vi "Command Editor Dialog 3.vi"(7 "Name(\"\" to use uuid)":string="Event CSM Tiny", 8 "Error in":errorcluster caption="Error in (no error)", 11 "CSM States":string="UI: Front Panel State >> Open -@ abc") -> (0 "Error out":errorcluster, 3 "Command out":string)   [LabVIEW 2017]
uses:
  _Shared/Single-Line Type.ctl
  _Shared/CSM Part Property.ctl
  _Shared/Single-Line Selection Type.ctl
  <vilib>/Utility/miscctls.llb/LVRowAndColumnUnsignedTypeDef.ctl
  AdvanceAPI/CSM - Keywords.vi
  _Support/Common/Trim Single line Text.vi
  AdvanceAPI/CSM - Break Down Multiple States String.vi
  AdvanceAPI/CSM - Compact Multiple States.vi
  _Polymophic/CSM - Filter Duplicated Lines.vi
  Communicable State Machine.lvlib
  _Shared/CSM Shared.lvlib
panel:
  out "MsgType":string
  out "Selction":string
  out "SelType":string
  out "Ref-String":string
  in  "clear arguments":bool
  in  "->|":bool
  in  "->":bool
  in  "-@":bool
  in  "Candidates":i32(listbox)
  # "Flood of Events:\n\nPanel/Pane Size Event\nSlide/Knob... User Event by dragging\nNumeric Control Value Change Event by Arraw Button"
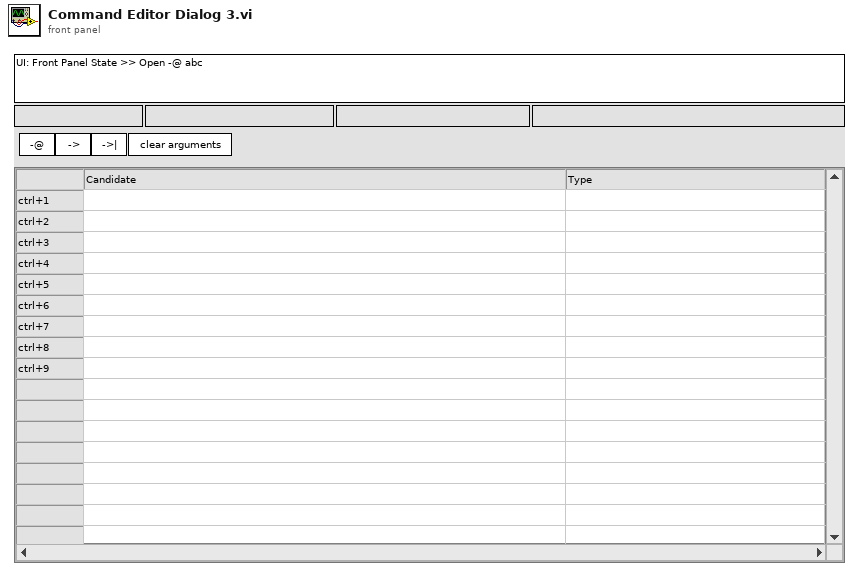
[diagram p1: front panel]
types:
  T1 = enum32{"Invalid", "Standard", "Closed", "Hidden", "Minimized", "Maximized"}
  T2 = enum32{"invalid app kind", "Development System", "Run Time System", "Student Edition", "Embedded LabVIEW", "Evaluation", "Custom"}
  T3 = typedef "LVRowAndColumnUnsignedTypeDef.ctl" = cluster{"Row":u32, "Column":u32}
  T4 = typedef "Communicable State Machine.lvlib/_CSM_Response Source Message.ctl" = cluster{"‘State":string, "’Arguments":string, "’Error":errorcluster}
  T5 = cluster{"Current VI Reference":refnum<vi>, "Close Panel on Exit?":bool}
  T6 = typedef "CSM Shared.lvlib/CSM Part Property.ctl" = cluster{"Section Start":u32, "Section End":u32, "Start":u32, "End":u32, "Section":string, "Core":string, "Sel Type":T7, "Ref-String":string}
  T7 = typedef "CSM Shared.lvlib/Single-Line Selection Type.ctl" = enum16{"<unknown>", "State-StateOrSignal", "State-ArgSymbol", "State-Arg", "Reg-Oper", "Reg-Symbol", "Msg-State", "Msg-Arg", "Msg-ArgSymbol", "Msg-Symbol", "Msg-Module", "Broadcast-Signal", "Broadcast-ArgSymbol", "Broadcast-Arg", "Broadcast-Symbol", "Broadcast-Oper", "Comment-Symbol", "Comment-Content"}
  T8 = typedef "CSM Shared.lvlib/Single-Line Type.ctl" = enum16{"State", "Message", "Broadcast", "Registration"}
  T9 = cluster{"Core":cluster{"Current VI Reference":refnum<vi>, "Close Panel on Exit?":bool}, "CSM States":string, "Selection":T6[], "Msg Type":T8}
  T10 = typedef "LVSelectionTypeDef.ctl" = cluster{"Selection Start":u32, "Selection End":u32}
  T11 = typedef "eventvkey.ctl" = enum16{"ASCII", "Enter", "Return", "Shift", "Ctrl", "Alt", "Cmd", "Opt", "Caps", "NumLock", "Clear", "Break", "Up", "Down", "Left", "Right", "Insert", "Delete", "Home", "End", "PageUp", "PageDown", "Escape", "Help", "Pause", "ScrollLock", "F1", "F2", "F3", "F4", "F5", "F6", "F7", "F8", "F9", "F10", "F11", "F12", "F13", "F14", "F15", "F16", "F17", "F18", "F19", "F20", "F21", "F22", "F23", "F24", "Play", "VolumeUp", "VolumeDown", "Mute", "Two Byte Char"}
  T12 = cluster{"Shift":bool, "Ctrl":bool, "Alt":bool, "Cmd":bool, "Opt":bool}
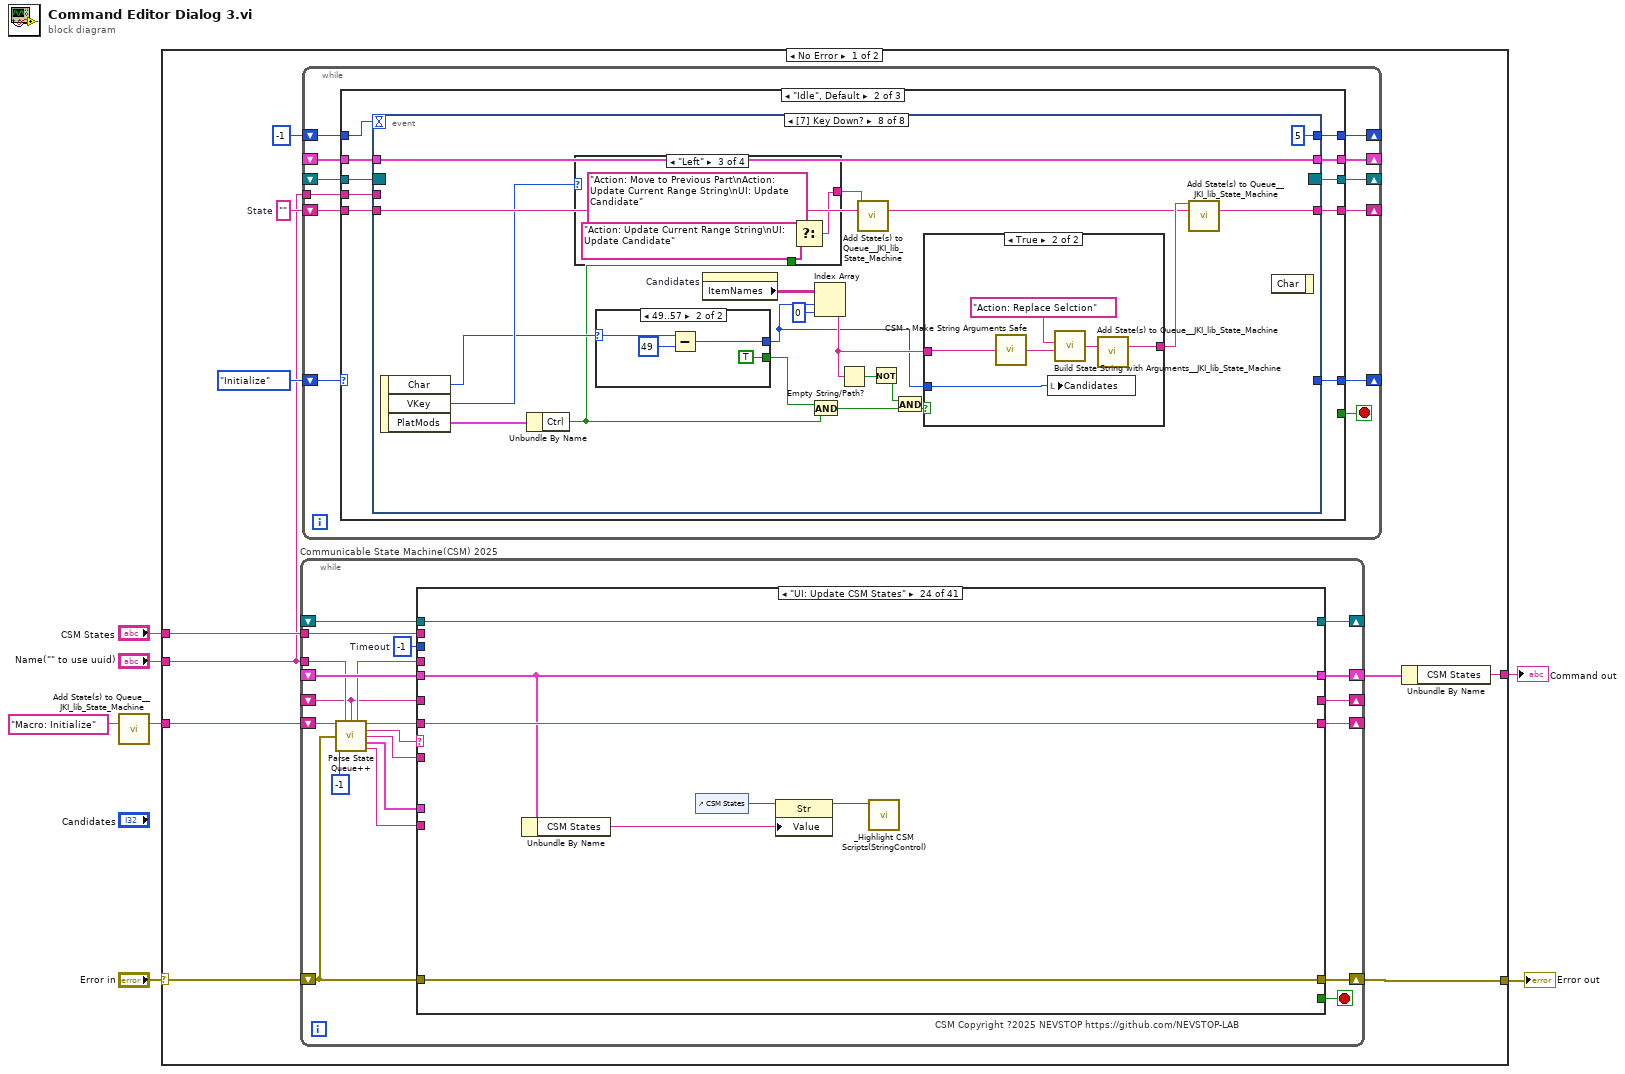
[diagram p0: block diagram]
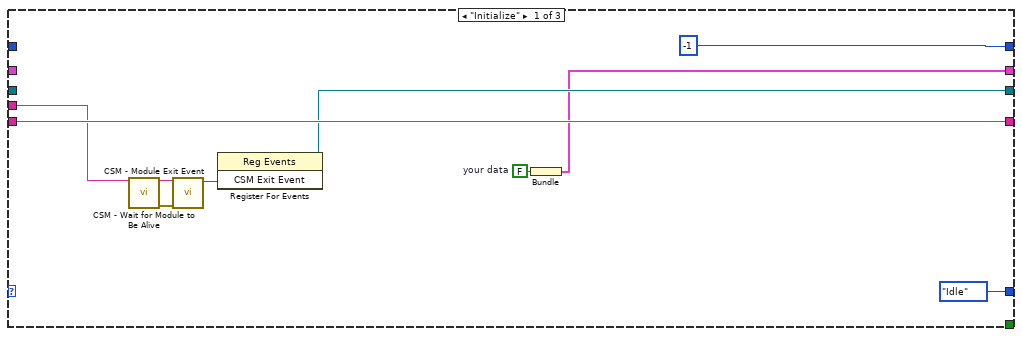
[diagram p2: hidden frame]
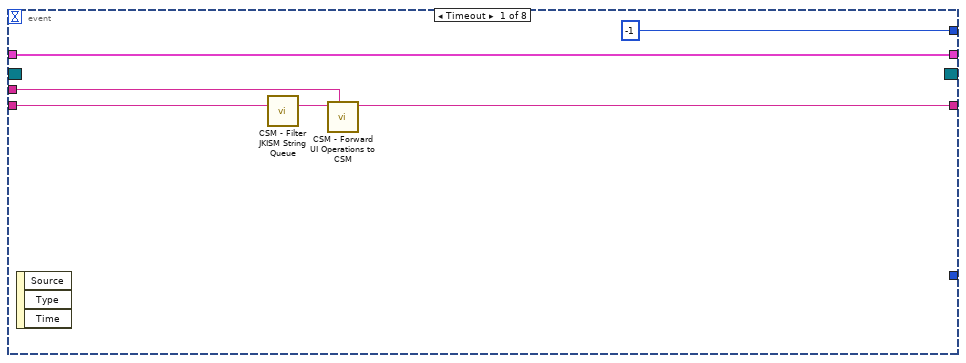
[diagram p3: hidden frame]
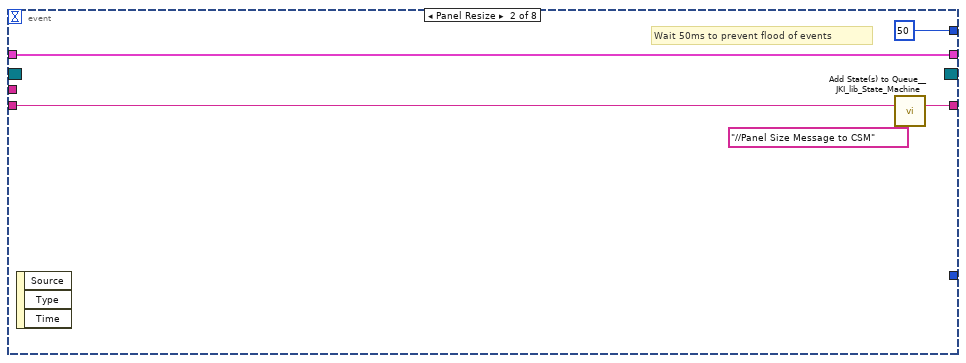
[diagram p4: hidden frame]
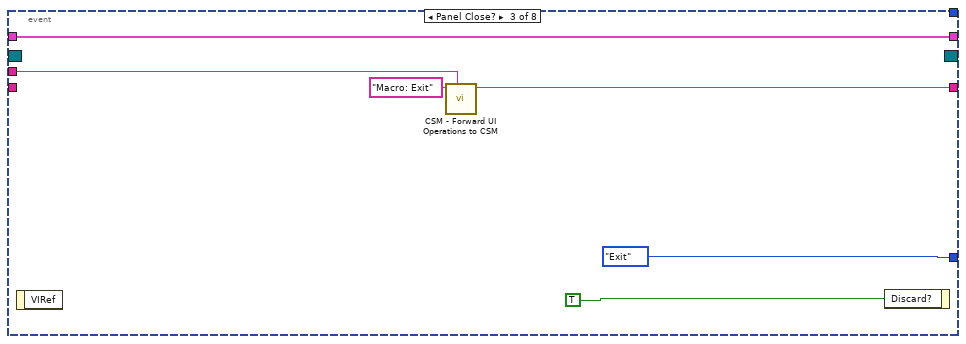
[diagram p5: hidden frame]
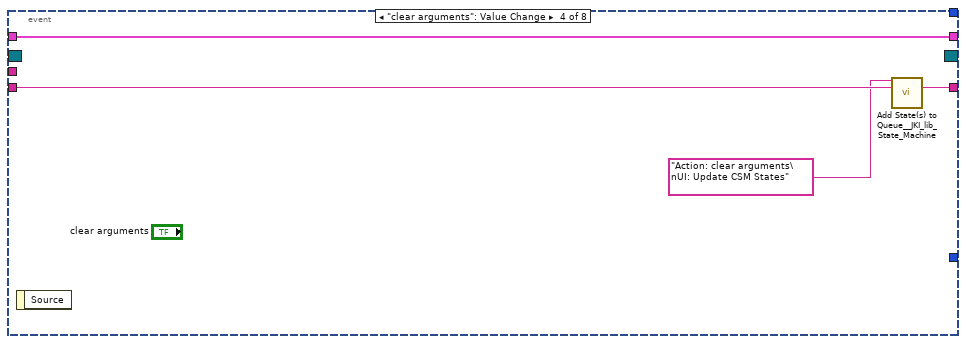
[diagram p6: hidden frame]
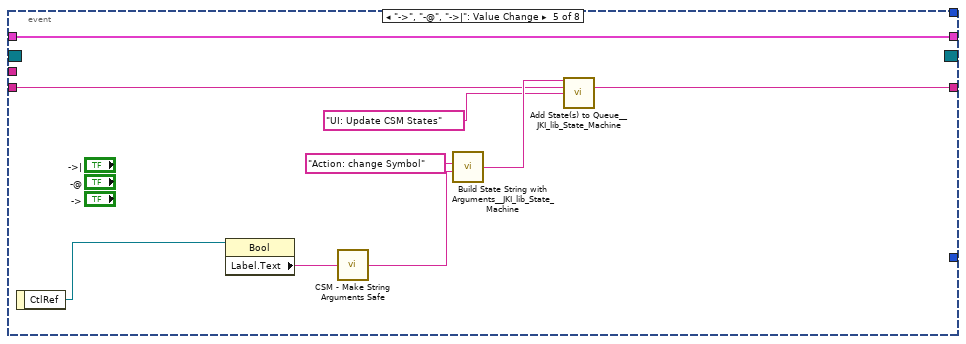
[diagram p7: hidden frame]
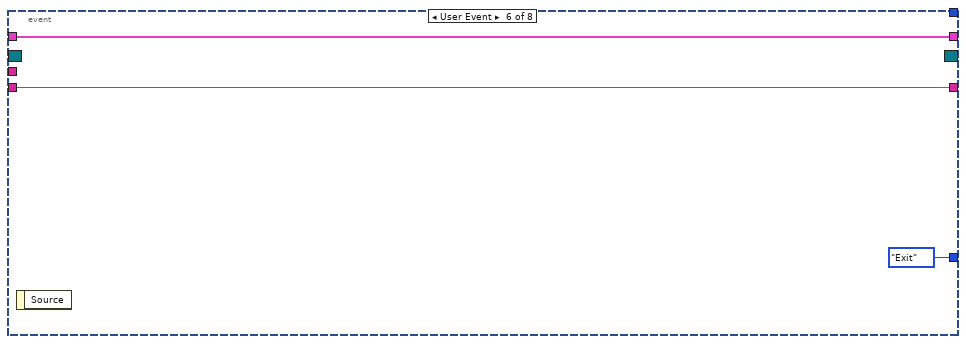
[diagram p8: hidden frame]
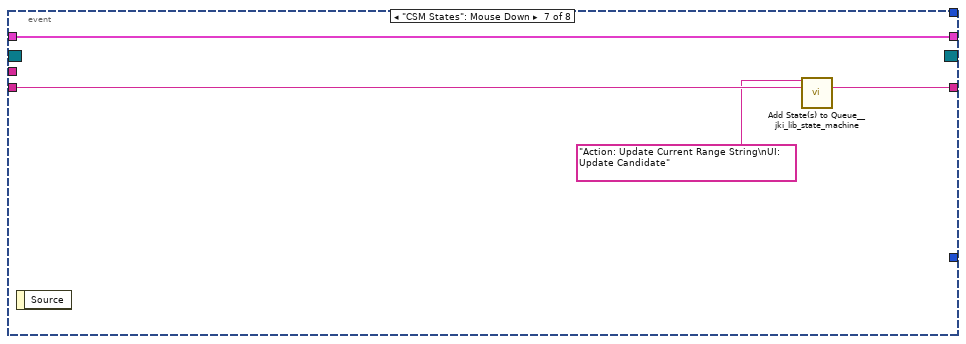
[diagram p9: hidden frame]
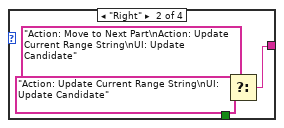
[diagram p11: hidden frame]
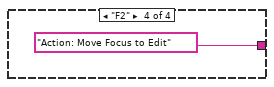
[diagram p12: hidden frame]
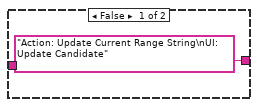
[diagram p13: hidden frame]
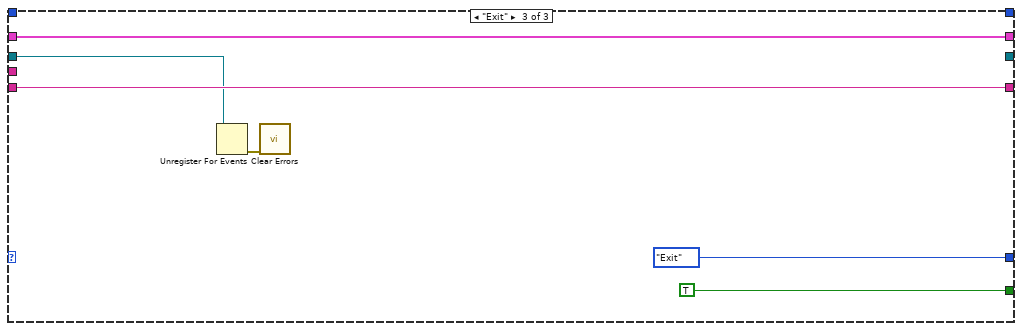
[diagram p15: hidden frame]
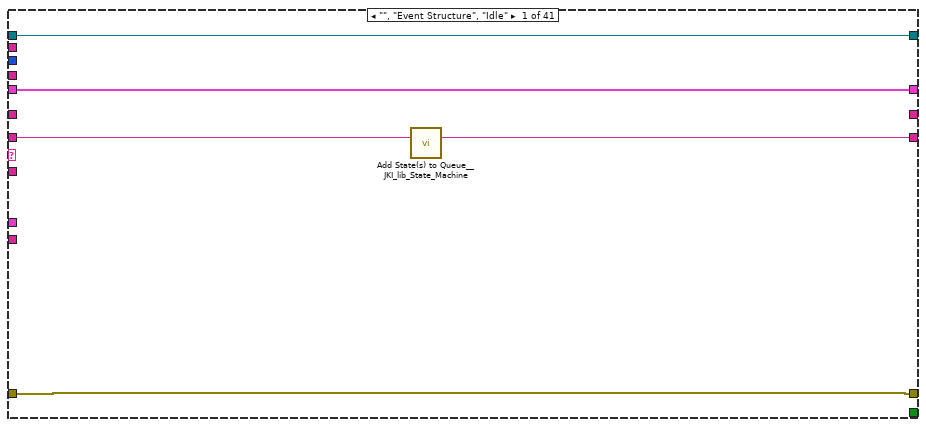
[diagram p16: hidden frame]
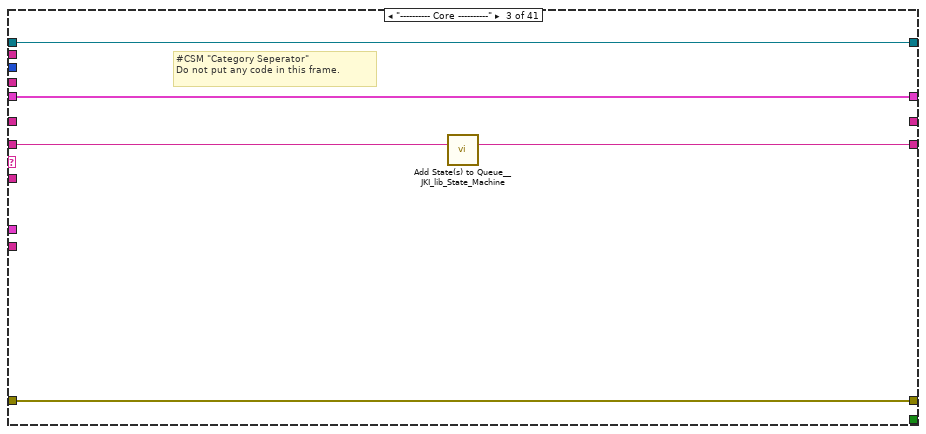
[diagram p18: hidden frame]
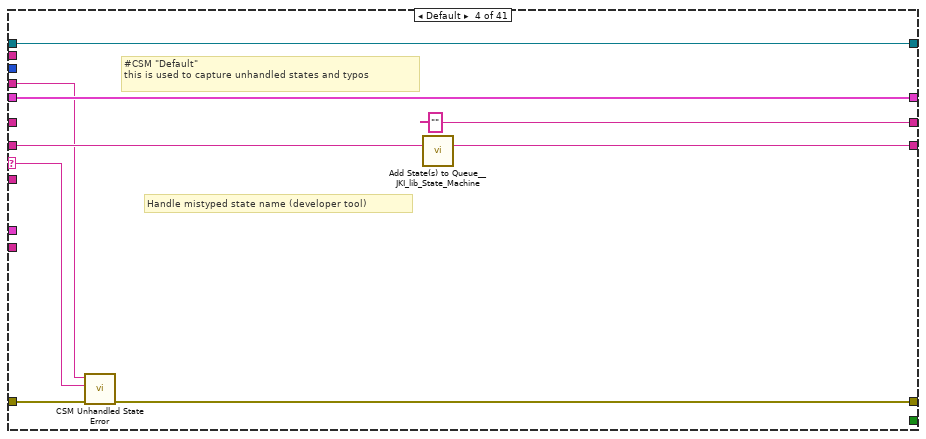
[diagram p19: hidden frame]
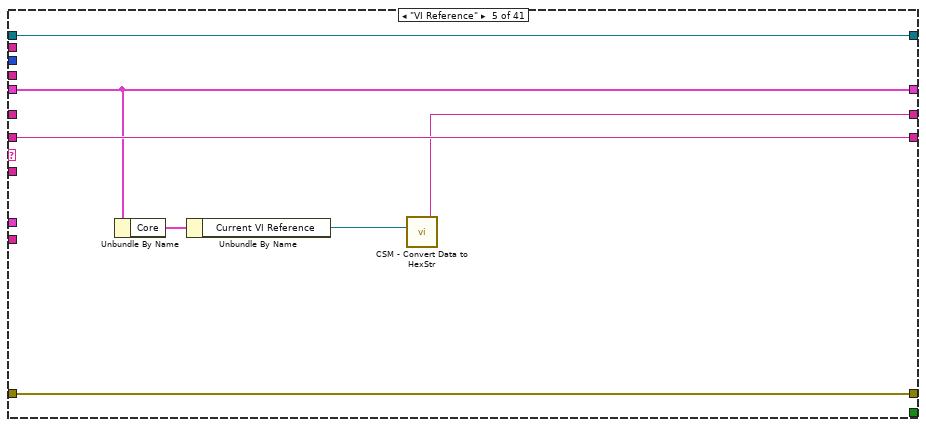
[diagram p20: hidden frame]
diagram:
  n1 = call <vilib>:"Add State(s) to Queue__JKI_lib_State_Machine.vi"("State(s) in (\"\")"="Macro: Initialize" ("Init State(\"Macro: Initialize\")")) -> ("States Out"=w7:string)  [unwired: 14 in]
  n2 = case shown="No Error" "Error in" {
    selector: "Error in" -> [w15 w645]
    tunnel: w7 -> [w17 _]
    tunnel: "Name(\"\" to use uuid)" -> [w8 _]
    tunnel: [w16 w645] -> w4
    tunnel: [w13 w644] -> w1
    tunnel: "CSM States" -> [w9 w644]
    frame No Error {
      w11 = ""  # State
      n3 = while "Communicable State Machine(CSM) 2025" {
        shift-right: [w148] -> w14
        shift-left: _ -> [w147]
        shift-right: [w151] -> w16
        shift-left: w15 -> [w145]
        shift-right: [w150] -> _
        shift-left: w17 -> [w152]
        tunnel: w8 -> [w141]
        shift-right: [w144] -> _
        shift-left: _ -> [w135]
        shift-right: [w143] -> _
        shift-left: _ -> [w142]
        tunnel: w9 -> [w134]
        stop <- w149 stop-if-true
        w146 = -1  # Timeout
        # "CSM Copyright ?2025 NEVSTOP https://github.com/NEVSTOP-LAB"
        n4 = call "Parse State Queue++.vi"("State Queue"=w152, "Name(\"\" to use uuid)"=w141, "Response Arguments"=w135, "Previous Error"=w145, "Dequeue Timeout(0ms)"=-1) -> ("Name Used"=w136:string, "Remaining States"=w153:string, "Current State"=w140:string, "Arguments"=w139:string, ">> Response Source Message >>"=w138:T4, ">> Source CSM >>"=w137:string)  [unwired: 5 in]
        n5 = case shown="\"UI: Update CSM States\"" w140 {
          selector: w140 -> [_ _ _ w170 _ _ _ _ _ _ _ _ _ _ _ _ _ _ _ _ _ _ _ _ _ _ _ _ _ _ _ _ _ _ _ _ _ _ _ _ _]
          tunnel: w153 -> [w154 w161 w167 w175 w182 w188 w211 w217 w224 w233 w246 w261 w267 w272 w281 w288 w293 w300 w304 w310 w318 w329 w345 w416 w420 w424 w435 w449 w455 w467 w470 w473 w485 w494 w514 w542 w571 w588 w593 w602 w627]
          tunnel: w139 -> [_ _ _ _ _ w187 w206 w216 w223 w232 _ _ _ _ _ _ _ _ _ _ _ w324 w339 _ _ _ _ _ _ _ _ w475 _ w486 w504 _ w565 _ _ _ _]
          tunnel: w147 -> [w156 w160 w164 w173 w181 w192 w212 w219 w226 w235 w245 w254 w265 w269 _ w283 w290 w299 w303 w307 w314 w327 w341 w414 w419 w423 w431 w446 w452 w464 w469 w479 w482 w492 w512 w540 w553 w582 w592 w601 w626]
          tunnel: [w157 w162 w165 w168 w183 errorcluster {"status"=FALSE, "code"=0, "source"=""} ("error out") w207 w214 w221 w238 w247 w258 w264 w270 w278 w284 w291 w294 w302 w308 w316 w325 w342 w417 w421 w425 w436 w447 w453 w465 w471 w480 w483 w495 w515 w543 w572 w589 w594 w603 w628] -> w151
          tunnel: w145 -> [w157 w162 w165 w176 w183 w189 w213 w215 w222 _ w247 w258 w264 w270 w278 w285 w291 _ w305 w308 w316 w326 w343 w417 w421 w425 w436 w447 w453 w465 w471 w480 w483 w495 w515 w543 w572 w589 w594 w603 w628]
          tunnel: [w158 w161 w166 w174 w182 w184 w210 w220 w227 w234 w246 w260 w266 w271 w280 w287 w292 w300 w304 w309 w317 w328 w344 w416 w420 w424 w435 w448 w454 w466 w470 w474 w484 w494 w514 w542 w571 w588 w593 w602 w627] -> w150
          tunnel: [_ _ _ _ _ _ TRUE _ _ _ _ _ TRUE _ _ _ _ _ _ _ _ _ _ _ _ _ _ _ _ _ _ _ _ _ _ _ _ _ _ _ _] -> w149
          tunnel: [w156 w160 w164 w173 w181 w192 w212 w219 w226 w236 w245 w259 w265 w269 w279 w283 w290 w299 w303 w307 w314 w327 w341 w414 w419 w423 w431 w446 w452 w464 w469 w477 w482 w489 w509 w537 w569 w581 w592 w601 w626] -> w148
          tunnel: w146 -> [_ _ _ _ _ _ _ _ _ _ _ _ _ _ _ _ _ _ _ _ _ _ _ _ _ _ _ _ _ _ _ _ _ _ _ _ _ _ _ _ _]
          tunnel: w137 -> [_ _ _ _ _ _ _ _ _ w230 _ _ _ _ _ _ _ _ _ _ _ _ _ _ _ _ _ _ _ _ _ _ _ _ _ _ _ _ _ _ _]
          tunnel: w138 -> [_ _ _ _ _ _ _ _ _ w237 _ _ _ _ _ _ _ _ _ _ _ _ _ _ _ _ _ _ _ _ _ _ _ _ _ _ _ _ _ _ _]
          tunnel: [_ _ _ "" w177 _ _ _ _ _ _ _ _ _ _ _ _ _ _ _ _ _ _ _ _ _ _ _ _ _ _ _ _ _ _ _ _ _ _ _ _] -> w144
          tunnel: [w155 w159 w163 w171 w180 w191 w208 w218 w225 w239 w244 w248 w262 w268 w276 w282 w289 w298 w301 w306 w315 w323 w338 w415 w418 w422 w434 w445 w450 w457 w468 w478 w481 w493 w513 w541 w570 w587 w591 w600 w625] -> w143
          tunnel: w142 -> [w155 w159 w163 w171 w180 w191 w208 w218 w225 w239 w244 w248 w262 w268 w276 w282 w289 _ w301 w306 w315 w323 w338 w415 w418 w422 w434 w445 w450 w457 w468 w478 w481 w493 w513 w541 w570 w587 w591 w600 w625]
          tunnel: w136 -> [_ _ _ w169 _ _ w205 _ _ _ _ _ _ _ _ _ _ w297 _ _ _ _ _ _ _ _ _ _ _ _ _ _ _ _ _ _ _ _ _ _ _]
          tunnel: w135 -> [_ _ _ _ _ _ _ _ _ _ _ _ _ _ _ _ _ _ _ _ _ _ _ _ _ _ _ _ _ _ _ _ _ _ _ _ _ _ _ _ _]
          tunnel: w134 -> [_ _ _ _ _ _ _ _ _ _ _ _ _ _ w275 _ _ _ _ _ _ _ _ _ _ _ _ _ _ _ _ _ _ _ _ _ _ _ _ _ _]
          frame "", "Event Structure", "Idle" {
            n6 = call <vilib>:"Add State(s) to Queue__JKI_lib_State_Machine.vi"("State(s) in (\"\")"=w154) -> ("States Out"=w158:string)  [unwired: 14 in]
          }
          frame "CSM Documentation" {
          }
          frame "---------- Core ----------" {
            # "#CSM \"Category Seperator\"\nDo not put any code in this frame."
            n7 = call <vilib>:"Add State(s) to Queue__JKI_lib_State_Machine.vi"("State(s) in (\"\")"=w167) -> ("States Out"=w166:string)  [unwired: 14 in]
          }
          frame Default {
            # "#CSM \"Default\"\nthis is used to capture unhandled states and typos"
            # "Handle mistyped state name (developer tool)"
            n8 = call "CSM Unhandled State Error.vi"("error in (no error)"=w176, "Current State"=w170, "CSM Name"=w169) -> ("error out"=w168:errorcluster)  [unwired: 8 in]
            n9 = call <vilib>:"Add State(s) to Queue__JKI_lib_State_Machine.vi"("State(s) in (\"\")"=w175) -> ("States Out"=w174:string)  [unwired: 14 in]
          }
          frame "VI Reference" {
            n10 = Unbundle By Name(w181) -> ("Core"=w179:T5)
            n11 = Unbundle By Name(w179) -> ("Current VI Reference"=w178:refnum<vi>)
            n12 = call "CSM - Convert Data to HexStr.vi"("Variant"=w178) -> ("HEX String (0-9,A-F)"=w177:string)  [unwired: 8 in]
          }
          frame "Error Handler" {
            # "#CSM Disable this error dialog if you need"
            # "#CSM \"Error Handler\"\nYou can also output any states to clean-up after errors occur"
            # "Clear error"
            n13 = case shown="Error" w189 {
              selector: w189 -> [_ w199]
              tunnel: [w198 w201] -> w185
              tunnel: w188 -> [w198 w200]
              tunnel: w187 -> [w197 _]
              tunnel: [w196 w199] -> w190
              frame No Error {
                n14 = call "CSM - Convert Argument to Error.vi"("Argument"=w197) -> ("error"=w196:errorcluster)  [unwired: 4 in]
                n15 = flat-sequence {
                  frame #0 {
                    # "#CSM External Error Handler Case\nUsually, it's because This CSM register others' \"Error Occurred\" status with \"Error Handler\". If other CSM have any error, the error will be passed here for central handling."
                  }
                }
              }
              frame Error {
                # "#CSM Internal Error Handler Case \nIf any error Occurred, \"Error Occurred\" \nstatus update will be broadcasted to system.\nParameter is Error Cluster."
                n16 = call "CSM - Convert Error to Argument.vi"("error"=w199) -> ("Argument"=w203:string)  [unwired: 4 in]
                n17 = call <vilib>:"Build State String with Arguments__JKI_lib_State_Machine.vi"("Arguments (\"\")"=w203, "State"="Error Occurred" ("Status with Arguments")) -> ("State with Arguments"=w202:string)  [unwired: 4 in]
                n18 = call "CSM - Broadcast Status Change.vi"("Status with Arguments"=w202, "State Queue"=w200) -> ("Remaining States"=w201:string)  [unwired: 13 in]
              }
            }
            n19 = disable-structure shown="Enabled" {
              disable-tunnel: w190 -> [w194 w195]
              frame Enabled {
                n20 = call <vilib>:"General Error Handler.vi"("error in (no error)"=w194) -> ()  [unwired: 10 in, 5 out]
              }
              frame Disabled {
                n21 = call <vilib>:"Clear Errors.vi"("error in (no error)"=w195) -> ()  [unwired: 5 in, 2 out]
              }
            }
            n22 = call <vilib>:"Add State(s) to Queue__JKI_lib_State_Machine.vi"("State(s) in Front (\"\")"="// Post Error States", "State(s) in (\"\")"=w185) -> ("States Out"=w184:string)  [unwired: 13 in]
          }
          frame "Critical Error" {
            # "#CSM Stop in Critical Error\nWhen Critical Error occurs, Stop the loop immediately. Do NOT change this unless you fully understand the impact."
            # "#CSM \"Critical Error\"\nWhen any un-recoverable error occurs, CSM goes into this case."
            n23 = call "CSM Critical Error.vi"("error in (no error)"=w213, "Arugments(as Reason)"=w206, "CSM Name"=w205) -> ("error out"=w207:errorcluster)  [unwired: 8 in]
            n24 = call <vilib>:"Add State(s) to Queue__JKI_lib_State_Machine.vi"("State(s) in (\"\")"=w211) -> ("States Out"=w210:string)  [unwired: 14 in]
          }
          frame "Target Error" {
            # "#CSM \"Target Error\"\nWhen This CSM try to communicate with an un-existed CSM, This CSM goes into this case."
            n25 = call "CSM Target Error.vi"("error in (no error)"=w215, "Arguments(as CSM Name)"=w216) -> ("error out"=w214:errorcluster)  [unwired: 9 in]
            n26 = call <vilib>:"Add State(s) to Queue__JKI_lib_State_Machine.vi"("State(s) in (\"\")"=w217) -> ("States Out"=w220:string)  [unwired: 14 in]
          }
          frame "Target Timeout Error" {
            # "#CSM \"Target Timeout Error\"\nWhen This CSM could not get the sync-call response in time, This CSM goes into this case."
            n27 = call "CSM Target Timeout Error.vi"("error in (no error)"=w222, "Arguments(as CSM Name)"=w223) -> ("error out"=w221:errorcluster)  [unwired: 9 in]
            n28 = call <vilib>:"Add State(s) to Queue__JKI_lib_State_Machine.vi"("State(s) in (\"\")"=w224) -> ("States Out"=w227:string)  [unwired: 14 in]
          }
          frame "Async Response", "Response" {
            n29 = Unbundle(w237) -> ("‘State"=w231:string, "’Arguments"=w229:string, "’Error"=w228:errorcluster)
            n30 = case shown="Default" w231 {
              tunnel: [w243] -> w238
              tunnel: w228 -> [w243]
              tunnel: [w242] -> w236
              tunnel: w235 -> [w242]
              tunnel: [w240] -> w234
              tunnel: w233 -> [w241]
              tunnel: w232 -> [_]
              tunnel: w230 -> [_]
              tunnel: w229 -> [_]
              frame Default {
                # "#CSM Response Comments\nAfter Message is executed, CSM goes to this state for receive the response.\n    For Async Message(->), \"Async Response\" is used. This CSM will goes to \"Async Message Posted\" immediately and receive the \"Async Response\" after the callee finishes the message.\n    For Sync Message(@),  This CSM will wait until the message is done and immediately goes to \"Response\""
                # "#CSM \"Async Response\"\nHandle Async-call Response (\"Async Response\" for ->)"
                # "#CSM \"Response\"\nHandle Sync-call Response (\"Response\" for -@)"
                n31 = call <vilib>:"Add State(s) to Queue__JKI_lib_State_Machine.vi"("State(s) in (\"\")"=w241) -> ("States Out"=w240:string)  [unwired: 14 in]
              }
            }
          }
          frame "Async Message Posted" {
            # "#CSM \"Async Message Posted\"\nAfter Async Message is posted (-> or ->| ), CSM goes to this state for post-action.\nYou can use Argument - State to tell which Async Message is called."
          }
          frame "Initialize Core Data" {
            # "#CSM \"Initialize Core Data\"\nThis is used to determine panel behavior on exit"
            # "originally closed?"
            # "exe?"
            # "If panel starts closed or is an EXE, then close it when we exit"
            n32 = property class="VI"() -> ("FP.State"=w251:T1)  [unwired: 2 in, 2 out]
            n33 = property class="App"() -> ("App.Kind"=w257:T2)  [unwired: 2 in, 2 out]
            n34 = control-ref of="Current VI Reference"() -> (w252:refnum<vi>)
            n35 = Equal?(x=w251, y=T1."Closed" ("Front Panel Window:State")) -> (x = y?=w249:bool)
            n36 = Equal?(x=w257, y=T2."Run Time System" ("Application:Kind")) -> (x = y?=w255:bool)
            n37 = Or(x=w249, y=w255) -> (x .or. y?=w253:bool)
            n38 = Bundle By Name(cluster=w254, "Core.Current VI Reference"=w252, "Core.Close Panel on Exit?"=w253) -> (w259:T9)
            n39 = call <vilib>:"Add State(s) to Queue__JKI_lib_State_Machine.vi"("State(s) in (\"\")"=w261) -> ("States Out"=w260:string)  [unwired: 14 in]
          }
          frame "Exit" {
            # "#CSM \"Exit\"\nCase for exiting the loop. No errors that occur here will be handled."
            n40 = call <vilib>:"Add State(s) to Queue__JKI_lib_State_Machine.vi"("State(s) in (\"\")"=w267) -> ("States Out"=w266:string)  [unwired: 14 in]
          }
          frame "---------- Data ----------" {
            # "#CSM \"Category Seperator\"\nDo not put any code in this frame."
            n41 = call <vilib>:"Add State(s) to Queue__JKI_lib_State_Machine.vi"("State(s) in (\"\")"=w272) -> ("States Out"=w271:string)  [unwired: 14 in]
          }
          frame "Data: Initialize" {
            w273 = T6[] []  # Selection
            w274 = Single-Line_Type."Registration"  # Msg Type
            w277 = T5 {"Current VI Reference"=refnum, "Close Panel on Exit?"=FALSE}  # Core
            n42 = call <vilib>:"Add State(s) to Queue__JKI_lib_State_Machine.vi"("State(s) in (\"\")"=w281) -> ("States Out"=w280:string)  [unwired: 14 in]
            n43 = Bundle("Core"=w277, "CSM States"=w275, "Selection"=w273, "Msg Type"=w274) -> (w279:T9)  [unwired: 1 in]
          }
          frame "Data: Cleanup" {
            # "Cleanup any data and references, here.\n(this is called automatically, by the Macro: Exit)"
            n44 = Unbundle By Name(w283) -> ("Core.Current VI Reference"=w286:refnum<vi>)
            n45 = Close Reference(reference=w286, error in (no error)=w285) -> (error out=w284:errorcluster)
            n46 = call <vilib>:"Add State(s) to Queue__JKI_lib_State_Machine.vi"("State(s) in (\"\")"=w288) -> ("States Out"=w287:string)  [unwired: 14 in]
          }
          frame "---------- Events ----------" {
            # "#CSM \"Category Seperator\"\nDo not put any code in this frame."
            n47 = call <vilib>:"Add State(s) to Queue__JKI_lib_State_Machine.vi"("State(s) in (\"\")"=w293) -> ("States Out"=w292:string)  [unwired: 14 in]
          }
          frame "Events: Register" {
            # "#CSM \"Events: Register\"\nRegister user event. New Message Event is registered to break CSM waiting in event structure by default."
            # "#CSM Register New Message Event\nRegister message event to break Waiting in Event structure."
            n48 = call "CSM - Get New State Notifier Event.vi"("Name(\"\" to use uuid) in"=w297) -> ("Error out"=w295:errorcluster, "New State Notifier Event"=w296:refnum<user-event>)  [unwired: 9 in]
            n49 = register-events(error in=w295, w296) -> (reference out=w298:refnum<event-registration>, error out=w294:errorcluster)  [unwired: 1 in]
          }
          frame "Events: Unregister" {
            # "#CSM \"Events: Unregister\"\nUnregister user event."
            n50 = Unregister For Events(event registration refnum=w301, error in=w305) -> (error out=w302:errorcluster)
          }
          frame "---------- UI ----------" {
            # "#CSM \"Category Seperator\"\nDo not put any code in this frame."
            n51 = call <vilib>:"Add State(s) to Queue__JKI_lib_State_Machine.vi"("State(s) in (\"\")"=w310) -> ("States Out"=w309:string)  [unwired: 14 in]
          }
          frame "UI: Initialize" {
            n52 = for {
              N: 9 -> [_]
              tunnel: [w320] -> w312 mode=indexing
              i -> [w322]
              n53 = Increment(x=w322) -> (x+1=w319:i32)
              n54 = Format Into String(format string="ctrl+%d", w319) -> (resulting string=w320:string)  [unwired: 2 in, 1 out]
            }
            n55 = property on="Candidates" class="MCListbox (strict)"("RowHdrs[]"=w312, "TopLeft"=T3 {"Row"=0, "Column"=0} ("Top Left Visible Cell")) -> ()  [unwired: 2 in, 2 out]
            n56 = call <vilib>:"Add State(s) to Queue__JKI_lib_State_Machine.vi"("State(s) in (\"\")"=w318) -> ("States Out"=w317:string)  [unwired: 14 in]
          }
          frame "UI: Cursor Set" {
            # "#CSM \"UI: Cursor Set\"\nSet and Unset Cursor Busy.\n(Usage: \"UI: Cursor Set >> Busy|Idle\")"
            # "Argument"
            n57 = disable-structure shown="Default" {
              disable-tunnel: w326 -> [w332 w337]
              disable-tunnel: [w331 w337] -> w325
              disable-tunnel: w324 -> [w330 _]
              frame condition #0 (active) {
                n58 = case shown="\"Idle\", Default" w330 {
                  tunnel: w332 -> [w334 w336]
                  tunnel: [w333 w335] -> w331
                  frame "Idle", Default {
                    n59 = call <vilib>:"Unset Busy.vi"("error in (no error)"=w334) -> ("error out"=w333:errorcluster)  [unwired: 10 in]
                  }
                  frame "Busy" {
                    n60 = call <vilib>:"Set Busy.vi"("error in (no error)"=w336) -> ("error out"=w335:errorcluster)  [unwired: 9 in, 1 out]
                  }
                }
              }
              frame condition #1 {
              }
            }
            n61 = call <vilib>:"Add State(s) to Queue__JKI_lib_State_Machine.vi"("State(s) in (\"\")"=w329) -> ("States Out"=w328:string)  [unwired: 14 in]
          }
          frame "UI: Front Panel State" {
            # "#CSM \"UI: Front Panel State\"\nSet Front Panel Open or Closed\n(Usage: \"UI: Front Panel State >> Open|Close\")"
            # "Argument"
            n62 = Unbundle By Name(w341) -> ("Core.Current VI Reference"=w340:refnum<vi>)
            n63 = call <vilib>:"Add State(s) to Queue__JKI_lib_State_Machine.vi"("State(s) in (\"\")"=w345) -> ("States Out"=w344:string)  [unwired: 14 in]
            n64 = case shown="\"Close\", \"Closed\"" w339 {
              tunnel: w343 -> [w351 w366 w377 w390 w403]
              tunnel: [w353 w367 w379 w392 w405] -> w342
              tunnel: w340 -> [w352 w364 w378 w391 w404]
              frame "Open", "Standard", Default {
                w346 = T1."Standard" ("State")
                n65 = property class="VI"(reference=w352, error in=w351) -> (reference out=w349:refnum<vi>, error out=w350:errorcluster, "FP.State"=w348:T1)
                n66 = Not Equal?(x=w348, y=w346) -> (x != y?=w347:bool)
                n67 = case shown="True" w347 {
                  tunnel: [w357 w359] -> w353
                  tunnel: w350 -> [w356 w359]
                  tunnel: w349 -> [w355 _]
                  tunnel: w346 -> [w354 _]
                  frame True {
                    n68 = invoke class="VI" method="FP.Open"(reference=w355, error in=w356, "Activate"=TRUE, "State"=w354) -> (error out=w357:errorcluster)  [unwired: 1 in, 4 out]
                  }
                  frame False {
                  }
                }
              }
              frame "Close", "Closed" {
                n69 = property class="VI"(reference=w364, error in=w366) -> (reference out=w363:refnum<vi>, error out=w365:errorcluster, "FP.State"=w361:T1)
                n70 = Not Equal?(x=w361, y=T1."Closed" ("Front Panel Window:State")) -> (x != y?=w360:bool)
                n71 = case shown="False" w360 {
                  tunnel: [w368 w371] -> w367
                  tunnel: w365 -> [w368 w370]
                  tunnel: w363 -> [_ w369]
                  frame False {
                  }
                  frame True {
                    n72 = invoke class="VI" method="FP.Close"(reference=w369, error in=w370) -> (error out=w371:errorcluster)  [unwired: 1 in, 2 out]
                  }
                }
              }
              frame "Hidden", "Hide" {
                w372 = T1."Hidden" ("State")
                n73 = property class="VI"(reference=w378, error in=w377) -> (reference out=w375:refnum<vi>, error out=w376:errorcluster, "FP.State"=w374:T1)
                n74 = Not Equal?(x=w374, y=w372) -> (x != y?=w373:bool)
                n75 = case shown="True" w373 {
                  tunnel: [w383 w384] -> w379
                  tunnel: w376 -> [w382 w384]
                  tunnel: w375 -> [w381 _]
                  tunnel: w372 -> [w380 _]
                  frame True {
                    n76 = invoke class="VI" method="FP.Open"(reference=w381, error in=w382, "State"=w380) -> (error out=w383:errorcluster)  [unwired: 2 in, 4 out]
                  }
                  frame False {
                  }
                }
              }
              frame "Minimize", "Minimized" {
                w385 = T1."Minimized" ("State")
                n77 = property class="VI"(reference=w391, error in=w390) -> (reference out=w388:refnum<vi>, error out=w389:errorcluster, "FP.State"=w387:T1)
                n78 = Not Equal?(x=w387, y=w385) -> (x != y?=w386:bool)
                n79 = case shown="True" w386 {
                  tunnel: [w396 w397] -> w392
                  tunnel: w389 -> [w395 w397]
                  tunnel: w388 -> [w394 _]
                  tunnel: w385 -> [w393 _]
                  frame True {
                    n80 = invoke class="VI" method="FP.Open"(reference=w394, error in=w395, "State"=w393) -> (error out=w396:errorcluster)  [unwired: 2 in, 4 out]
                  }
                  frame False {
                  }
                }
              }
              frame "Maximize", "Maximized" {
                w398 = T1."Maximized" ("State")
                n81 = property class="VI"(reference=w404, error in=w403) -> (reference out=w401:refnum<vi>, error out=w402:errorcluster, "FP.State"=w400:T1)
                n82 = Not Equal?(x=w400, y=w398) -> (x != y?=w399:bool)
                n83 = case shown="True" w399 {
                  tunnel: [w409 w410] -> w405
                  tunnel: w402 -> [w408 w410]
                  tunnel: w401 -> [w407 _]
                  tunnel: w398 -> [w406 _]
                  frame True {
                    n84 = invoke class="VI" method="FP.Open"(reference=w407, error in=w408, "State"=w406) -> (error out=w409:errorcluster)  [unwired: 2 in, 4 out]
                  }
                  frame False {
                  }
                }
              }
            }
          }
          frame "UI: Update CSM States" {
            n85 = Unbundle By Name(w414) -> ("CSM States"=w412:string)
            n86 = control-ref of="CSM States"() -> (w413:refnum<vi>)
            n87 = property class="Str"(reference=w413, "Value"=w412) -> (reference out=w411:refnum<vi>)  [unwired: 1 in, 1 out]
            n88 = call "_Highlight CSM Scripts(StringControl).vi"("String Ctrl"=w411) -> ()  [unwired: 10 in, 1 out]
          }
          frame "UI: Update CSM Candidates" {
          }
          frame "UI: Update CSM-VI Candidates" {
          }
          frame "UI: Update Candidate" {
            n89 = Unbundle By Name(w431) -> ("Selection"=w430:T6[])
            n90 = for {
              tunnel: w430 -> [w444] mode=indexing
              tunnel: [w437] -> w427 mode=concatenating
              tunnel: [w438] -> w426 mode=concatenating
              n91 = Unbundle By Name(w444) -> ("Sel Type"=w443:T7)
              n92 = call "_scriptEditor.Input Candidates.vi"("Selection"=w444) -> ("Array"=w438:string[])  [unwired: 10 in]
              n93 = Format Into String(w443) -> (resulting string=w442:string)  [unwired: 3 in, 1 out]
              n94 = Array Size(array=w438) -> (size(s)=w441:i32)
              n95 = Initialize Array(w442, w441) -> (w440:string[])
              n96 = Build Array(w438, w440) -> (w439:string[][])
              n97 = Transpose 2D Array(2D array=w439) -> (transposed array=w437:string[][])
            }
            n98 = Index Array(array=w430) -> (element=w429:T6)  [unwired: 1 in]
            n99 = Unbundle By Name(w429) -> ("Section"=w428:string)
            n100 = call <vilib>:"Trim Whitespace.vi"("string"=w428) -> ("trimmed string"=w433:string)  [unwired: 1 in]
            n101 = Search 1D Array(1D array=w426, element=w433) -> (index of element=w432:i32)  [unwired: 1 in]
            n102 = property on="Candidates" class="MCListbox (strict)"("ItemNames"=w427, "Value"=w432) -> ()  [unwired: 2 in, 2 out]
          }
          frame "---------- Macro ----------" {
            # "#CSM \"Category Seperator\"\nDo not put any code in this frame."
            n103 = call <vilib>:"Add State(s) to Queue__JKI_lib_State_Machine.vi"("State(s) in (\"\")"=w449) -> ("States Out"=w448:string)  [unwired: 14 in]
          }
          frame "Macro: Initialize" {
            # "#CSM \"Macro: Initialize\"\nInitialization Macro (This is called once, when the VI starts)"
            n104 = call <vilib>:"Add State(s) to Queue__JKI_lib_State_Machine.vi"("State(s) in Front (\"\")"="Data: Initialize\nInitialize Core Data\nEvents: Register\nUI: Initialize\n//UI: Front Panel State >> Open\nUI: Update CSM States", "State(s) in (\"\")"=w455) -> ("States Out"=w454:string)  [unwired: 13 in]
          }
          frame "Macro: Exit" {
            # "#CSM \"Macro: Exit\"\nExit Macro (This is called once, when the VI exits)"
            n105 = Unbundle By Name(w464) -> ("Core.Close Panel on Exit?"=w463:bool)
            n106 = Select(t="UI: Front Panel State >> Close", s=w463, f="") -> (s? t:f=w460:string)
            n107 = call <vilib>:"Add State(s) to Queue__JKI_lib_State_Machine.vi"("State(s) in Front (\"\")"="//Exit Sub-Modules ", "State(s) in (\"\")"=w460, "State(s) at Back (\"\")"="Data: Cleanup\nEvents: Unregister\nExit") -> ("States Out"=w458:string)  [unwired: 12 in]
            n108 = call <vilib>:"Add State(s) to Queue__JKI_lib_State_Machine.vi"("State(s) in Front (\"\")"=w458, "State(s) in (\"\")"=w467) -> ("States Out"=w466:string)  [unwired: 13 in]
          }
          frame "---------- API ----------" {
            # "#CSM \"Category Seperator\"\nDo not put any code in this frame."
          }
          frame "API: Set Command" {
            # "#CSM API Example\nCopy/Rename this case for your own API"
            n109 = call "CSM - Revert Arguments-Safe String.vi"("Safe Argurment String"=w475) -> ("Origin Argurment String"=w476:string)  [unwired: 8 in]
            n110 = Bundle By Name(cluster=w479, "CSM States"=w476) -> (w477:T9)
            n111 = call <vilib>:"Add State(s) to Queue__JKI_lib_State_Machine.vi"("State(s) in (\"\")"=w473, "State(s) at Back (\"\")"="UI: Refresh Inputs" ("State(s) in Front (\"\")")) -> ("States Out"=w474:string)  [unwired: 13 in]
          }
          frame "---------- Action ----------" {
            # "#CSM \"Category Seperator\"\nDo not put any code in this frame."
            n112 = call <vilib>:"Add State(s) to Queue__JKI_lib_State_Machine.vi"("State(s) in (\"\")"=w485) -> ("States Out"=w484:string)  [unwired: 14 in]
          }
          frame "Action: Change Comments" {
            n113 = Unbundle By Name(w492) -> ("CSM States"=w491:string)
            n114 = Match Pattern(string=w491, regular expression="//") -> (before substring=w488:string)  [unwired: 1 in, 3 out]
            n115 = call "Build State String with Comments.vi"("Comments"=w486, "State"=w488) -> ("State with Arguments"=w487:string)  [unwired: 6 in]
            n116 = Bundle By Name(cluster=w492, "CSM States"=w487) -> (w489:T9)
          }
          frame "Action: change Symbol" {
            w499 = " " ("regular expression")
            n117 = Unbundle By Name(w512) -> ("CSM States"=w511:string)
            n118 = Match Pattern(string=w511, regular expression="//") -> (before substring=w507:string, after substring=w508:string)  [unwired: 1 in, 2 out]
            n119 = for {
              tunnel: w507 -> [w522]
              tunnel: string[] ["->|", "-@", "->"] ("regular expression") -> [w521] mode=indexing
              tunnel: [w519] -> _ if=w518
              tunnel: [w517] -> w505
              tunnel: [w516] -> w500
              stop <- w518 stop-if-true
              n120 = Match Pattern(string=w522, regular expression=w521) -> (before substring=w517:string, match substring=w519:string, after substring=w516:string, offset past match=w520:i32)  [unwired: 1 in]
              n121 = Greater Or Equal To 0?(x=w520) -> (x >= 0?=w518:bool)
            }
            n122 = call "CSM - Revert Arguments-Safe String.vi"("Safe Argurment String"=w504) -> ("Origin Argurment String"=w503:string)  [unwired: 8 in]
            n123 = call <vilib>:"Trim Whitespace.vi"("string"=w505) -> ("trimmed string"=w502:string)  [unwired: 1 in]
            n124 = call <vilib>:"Trim Whitespace.vi"("string"=w500) -> ("trimmed string"=w501:string)  [unwired: 1 in]
            n125 = call <vilib>:"Trim Whitespace.vi"("string"=w508) -> ("trimmed string"=w496:string)  [unwired: 1 in]
            n126 = Concatenate Strings(w502, w499, w503, w499, w501) -> (w497:string)
            n127 = call "Build State String with Comments.vi"("Comments"=w496, "State"=w497) -> ("State with Arguments"=w498:string)  [unwired: 6 in]
            n128 = Bundle By Name(cluster=w512, "CSM States"=w498) -> (w509:T9)
          }
          frame "Action: clear arguments" {
            w533 = " " ("regular expression")
            n129 = Unbundle By Name(w540) -> ("CSM States"=w539:string)
            n130 = Match Pattern(string=w539, regular expression="//") -> (before substring=w535:string, after substring=w536:string)  [unwired: 1 in, 2 out]
            n131 = for {
              tunnel: w535 -> [w550]
              tunnel: string[] ["->|", "-@", "->"] ("regular expression") -> [w549] mode=indexing
              tunnel: [w547] -> w529 if=w546
              tunnel: [w545] -> w531
              tunnel: [w544] -> w524
              stop <- w546 stop-if-true
              n132 = Match Pattern(string=w550, regular expression=w549) -> (before substring=w545:string, match substring=w547:string, after substring=w544:string, offset past match=w548:i32)  [unwired: 1 in]
              n133 = Greater Or Equal To 0?(x=w548) -> (x >= 0?=w546:bool)
            }
            n134 = call <vilib>:"Trim Whitespace.vi"("string"=w536) -> ("trimmed string"=w526:string)  [unwired: 1 in]
            n135 = Match Pattern(string=w531, regular expression=">>") -> (before substring=w525:string)  [unwired: 1 in, 3 out]
            n136 = call <vilib>:"Trim Whitespace.vi"("string"=w524) -> ("trimmed string"=w523:string)  [unwired: 1 in]
            n137 = call <vilib>:"Build State String with Arguments__JKI_lib_State_Machine.vi"("State"=w525) -> ("State with Arguments"=w530:string)  [unwired: 5 in]
            n138 = Concatenate Strings(w530, w533, w529, w533, w523) -> (w527:string)
            n139 = call "Build State String with Comments.vi"("Comments"=w526, "State"=w527) -> ("State with Arguments"=w528:string)  [unwired: 6 in]
            n140 = Bundle By Name(cluster=w540, "CSM States"=w528) -> (w537:T9)
          }
          frame "Action: Replace Selction" {
            n141 = Unbundle By Name(w553) -> ("Selection"=w552:T6[])
            n142 = Index Array(array=w552) -> (element=w551:T6)  [unwired: 1 in]
            n143 = property on="CSM States" class="Str"() -> ("Value"=w564:string)  [unwired: 2 in, 2 out]
            n144 = Unbundle By Name(w551) -> ("Start"=w567:u32, "End"=w568:u32)
            n145 = Subtract(x=w568, y=w567) -> (x-y=w566:u32)
            n146 = call "CSM - Revert Arguments-Safe String.vi"("Safe Argurment String"=w565) -> ("Origin Argurment String"=w559:string)  [unwired: 8 in]
            n147 = control-ref of="CSM States"() -> (w562:refnum<vi>)
            n148 = Replace Substring(2:w566, 3:w567, 4:w559, 5:w564) -> (1:w558:string)  [unwired: 1 out]
            n149 = property class="Str"(reference=w562, "Value"=w558) -> (reference out=w556:refnum<vi>)  [unwired: 1 in, 1 out]
            n150 = String Length(string=w558) -> (length=w557:i32)
            n151 = Search/Split String(string=w558, search string/char (-)=w559) -> (substring before match=w560:string, match + rest of string=w561:string, offset of match=w554:i32)  [unwired: 1 in]
            n152 = String Length(string=w559) -> (length=w563:i32)
            n153 = Add(x=w554, y=w563) -> (x+y=w555:i32)
            n154 = call "_Highlight CSM Scripts(StringControl).vi"("String Ctrl"=w556) -> ()  [unwired: 10 in, 1 out]
            n155 = flat-sequence {
              tunnel: w561 -> [_]
              tunnel: w560 -> [_]
              tunnel: w557 -> [_]
              frame #0 {
              }
            }
            n156 = Bundle By Name(cluster=w553, "Msg Type"=w555, "CSM States"=w558) -> (w569:T9)
          }
          frame "Action: Update Current Range String" {
            n157 = control-ref of="CSM States"() -> (w585:refnum<vi>)
            n158 = property class="Str"(reference=w585) -> ("Value"=w586:string, "Text.Selection"=w584:T10)  [unwired: 1 in, 2 out]
            n159 = Unbundle By Name(w584) -> ("Selection Start"=w583:u32)
            n160 = call "CSM Part Property at Cursor.vi"("Pos"=w583, "single-line text"=w586) -> ("Msg Type"=w580:T8, "Property"=w573:T6[])  [unwired: 7 in, 1 out]
            n161 = Index Array(array=w573) -> (element=w577:T6)  [unwired: 1 in]
            n162 = Unbundle By Name(w577) -> ("Section"=→"Selction":string, "Sel Type"=w575:T7, "Ref-String"=→"Ref-String":string)
            n163 = Bundle By Name(cluster=w582, "Selection"=w573, "Msg Type"=w580) -> (w581:T9)
            n164 = Format Into String(w580) -> (resulting string=→"MsgType":string)  [unwired: 3 in, 1 out]
            n165 = Format Into String(w575) -> (resulting string=→"SelType":string)  [unwired: 3 in, 1 out]
          }
          frame "Action: Move Focus to Edit" {
            n166 = property on="CSM States" class="Str"("Key Focus"=TRUE) -> ()  [unwired: 2 in, 2 out]
          }
          frame "Action: Move to Next Part" {
            n167 = property on="CSM States" class="Str"() -> ("Value"=w596:string, "Key Focus"=w599:bool, "Text.Selection End"=w598:u32, "Text.Selection Start"=w597:u32)  [unwired: 2 in, 2 out]
            n168 = Max & Min(x=w598, y=w597) -> (min(x,y)=w595:u32)  [unwired: 1 out]
            n169 = case shown="True" w599 {
              tunnel: w596 -> [_ w611]
              tunnel: w595 -> [_ w610]
              frame False {
              }
              frame True {
                n170 = call "Single-Line To CSM Parts.vi"("single-line text"=w611) -> ("Property"=w609:T6[])  [unwired: 7 in, 3 out]
                n171 = for {
                  tunnel: w610 -> [w619]
                  tunnel: w609 -> [w614] mode=indexing
                  tunnel: [w614] -> _ mode=indexing if=w612
                  tunnel: [w613] -> w608 mode=indexing if=w612
                  i -> [w613]
                  n172 = Unbundle By Name(w614) -> ("Section Start"=w615:u32, "Section End"=w616:u32)
                  n173 = Greater Or Equal?(x=w619, y=w615) -> (x >= y?=w617:bool)
                  n174 = Less Or Equal?(x=w619, y=w616) -> (x <= y?=w618:bool)
                  n175 = And(x=w618, y=w617) -> (x .and. y?=w612:bool)
                }
                n176 = Array Max & Min(array=w608) -> (max value=w607:i32)  [unwired: 3 out]
                n177 = Increment(x=w607) -> (x+1=w606:i32)
                n178 = Index Array(array=w609, index=w606) -> (element=w605:T6)
                n179 = Unbundle By Name(w605) -> ("Start"=w604:u32)
                n180 = property on="CSM States" class="Str"("Text.Selection End"=w604, "Text.Selection Start"=w604) -> ()  [unwired: 2 in, 2 out]
              }
            }
          }
          frame "Action: Move to Previous Part" {
            n181 = property on="CSM States" class="Str"() -> ("Value"=w621:string, "Key Focus"=w624:bool, "Text.Selection End"=w623:u32, "Text.Selection Start"=w622:u32)  [unwired: 2 in, 2 out]
            n182 = Max & Min(x=w623, y=w622) -> (min(x,y)=w620:u32)  [unwired: 1 out]
            n183 = case shown="True" w624 {
              tunnel: w621 -> [_ w635]
              tunnel: w620 -> [_ w634]
              frame False {
              }
              frame True {
                n184 = call "Single-Line To CSM Parts.vi"("single-line text"=w635) -> ("Property"=w633:T6[])  [unwired: 7 in, 3 out]
                n185 = for {
                  tunnel: w634 -> [w643]
                  tunnel: w633 -> [w638] mode=indexing
                  tunnel: [w638] -> _ mode=indexing if=w636
                  tunnel: [w637] -> w630 mode=indexing if=w636
                  i -> [w637]
                  n186 = Unbundle By Name(w638) -> ("Section Start"=w639:u32, "Section End"=w640:u32)
                  n187 = Greater Or Equal?(x=w643, y=w639) -> (x >= y?=w641:bool)
                  n188 = Less Or Equal?(x=w643, y=w640) -> (x <= y?=w642:bool)
                  n189 = And(x=w642, y=w641) -> (x .and. y?=w636:bool)
                }
                n190 = Array Max & Min(array=w630) -> (min value=w629:i32)  [unwired: 3 out]
                n191 = Index Array(array=w633, index=w629) -> (element=w632:T6)
                n192 = Unbundle By Name(w632) -> ("Start"=w631:u32)
                n193 = property on="CSM States" class="Str"("Text.Selection End"=w631, "Text.Selection Start"=w631) -> ()  [unwired: 2 in, 2 out]
              }
            }
          }
        }
      }
      n194 = while {
        shift-right: [w28] -> _
        shift-left: enum16{"Idle", "Initialize", "Exit"}."Initialize" -> [w29]
        tunnel: w8 -> [w26]
        shift-right: [w24] -> _
        shift-left: w11 -> [w25]
        shift-right: [w22] -> _
        shift-left: -1 -> [w23]
        shift-right: [w21] -> _
        shift-left: _ -> [w20]
        shift-right: [w19] -> _
        shift-left: _ -> [w18]
        stop <- w27 stop-if-true
        n195 = case shown="\"Idle\", Default" w29 {
          tunnel: [enum16{"Idle", "Initialize", "Exit"}."Idle" w49 enum16{"Idle", "Initialize", "Exit"}."Exit"] -> w28
          tunnel: [_ _ TRUE] -> w27
          tunnel: w26 -> [w35 w48 _]
          tunnel: w25 -> [w38 w46 w130]
          tunnel: [w38 w47 w130] -> w24
          tunnel: w23 -> [_ w44 _]
          tunnel: [-1 w45 _] -> w22
          tunnel: [w34 w42 _] -> w21
          tunnel: w20 -> [_ w43 w129]
          tunnel: [w30 w40 w127] -> w19
          tunnel: w18 -> [_ w41 w127]
          frame "Initialize" {
            w31 = FALSE  # your data
            n196 = call "CSM - Wait for Module to Be Alive.vi"("CSM Name"=w35) -> ("CSM Name(dup)"=w33:string, "error out"=w32:errorcluster)  [unwired: 12 in, 1 out]
            n197 = call "CSM - Module Exit Event.vi"("Error in"=w32, "Name(\"\" to use uuid) in"=w33) -> ("CSM Exit Event"=w36:refnum<user-event>)  [unwired: 8 in, 1 out]
            n198 = register-events(w36) -> (reference out=w34:refnum<event-registration>)  [unwired: 2 in, 1 out]
            n199 = Bundle("your data"=w31) -> (w30:cluster{"your data":bool})  [unwired: 1 in]
          }
          frame "Idle", Default {
            n200 = event shown="[7] Key Down?" {
              selector: w43 -> [_ _ _ _ _ _ _ _]
              dyn-events: [_ _ _ _ _ _ _ _] -> w42
              timeout: w44 -> [_ _ _ _ _ _ _ _]
              tunnel: [_ _ enum16{"Idle", "Initialize", "Exit"}."Exit" _ _ enum16{"Idle", "Initialize", "Exit"}."Exit" _ _] -> w49
              tunnel: w48 -> [w53 _ w63 _ _ _ _ _]
              tunnel: w46 -> [w51 w60 _ w68 w73 w82 w84 w93]
              tunnel: [w54 w59 w62 w69 w72 w82 w85 w92] -> w47
              tunnel: [-1 50 _ _ _ _ _ 5] -> w45
              tunnel: w41 -> [w52 w56 w61 w70 w79 w80 w86 w106]
              tunnel: [w52 w56 w61 w70 w79 w80 w86 w106] -> w40
              event Timeout {
                n201 = event-data() -> ()  [unwired: 1 in, 3 out]
                n202 = call-poly "CSM - Filter JKISM String Queue.vi"("State(s) in (\"\")"=w51) -> ("States Out"=w50:string)  [unwired: 14 in]
                n203 = call "CSM - Forward UI Operations to CSM.vi"("Name(\"\" to use uuid)"=w53, "State(s) in (\"\")"=w50) -> ("States Out"=w54:string)  [unwired: 9 in]
              }
              event Panel Resize {
                # "Wait 50ms to prevent flood of events"
                n204 = event-data() -> ()  [unwired: 1 in, 3 out]
                n205 = call <vilib>:"Add State(s) to Queue__JKI_lib_State_Machine.vi"("State(s) in (\"\")"=w60, "State(s) at Back (\"\")"="//Panel Size Message to CSM" ("State(s) at Back (\"\")")) -> ("States Out"=w59:string)  [unwired: 13 in]
              }
              event Panel Close? {
                n206 = event-data() -> ()  [unwired: 1 in, 1 out]
                n207 = call "CSM - Forward UI Operations to CSM.vi"("Name(\"\" to use uuid)"=w63, "State(s) in (\"\")"="Macro: Exit" ("State")) -> ("States Out"=w62:string)  [unwired: 9 in]
                n208 = event-data("Discard?"=TRUE) -> ()  [unwired: 1 in, 1 out]
              }
              event "clear arguments": Value Change {
                n209 = event-data() -> ()  [unwired: 1 in, 1 out]
                n210 = call <vilib>:"Add State(s) to Queue__JKI_lib_State_Machine.vi"("State(s) in Front (\"\")"="Action: clear arguments\nUI: Update CSM States" ("State(s) in Front (\"\")"), "State(s) in (\"\")"=w68) -> ("States Out"=w69:string)  [unwired: 13 in]
              }
              event "->", "-@", "->|": Value Change {
                n211 = event-data() -> ("CtlRef"=w71:refnum<vi>)  [unwired: 1 in]
                n212 = property class="Bool"(reference=w71) -> ("Label.Text"=w76:string)  [unwired: 1 in, 2 out]
                n213 = call "CSM - Make String Arguments Safe.vi"("Argurment String"=w76) -> ("Safe Argurment String"=w75:string)  [unwired: 8 in]
                n214 = call <vilib>:"Build State String with Arguments__JKI_lib_State_Machine.vi"("Arguments (\"\")"=w75, "State"="Action: change Symbol") -> ("State with Arguments"=w78:string)  [unwired: 4 in]
                n215 = call <vilib>:"Add State(s) to Queue__JKI_lib_State_Machine.vi"("State(s) in Front (\"\")"=w78, "State(s) in (\"\")"=w73, "State(s) at Back (\"\")"="UI: Update CSM States" ("State")) -> ("States Out"=w72:string)  [unwired: 12 in]
              }
              event User Event {
                n216 = event-data() -> ()  [unwired: 1 in, 1 out]
              }
              event "CSM States": Mouse Down {
                n217 = event-data() -> ()  [unwired: 1 in, 1 out]
                n218 = call <vilib>:"Add State(s) to Queue__jki_lib_state_machine.vi"("State(s) in Front (\"\")"="Action: Update Current Range String\nUI: Update Candidate" ("State(s) at Back (\"\")"), "State(s) in (\"\")"=w84) -> ("States Out"=w85:string)  [unwired: 13 in]
              }
              event Key Down? {
                n219 = event-data() -> ("Char"=w89:i16, "VKey"=w90:T11, "PlatMods"=w91:T12)  [unwired: 1 in]
                n220 = Unbundle By Name(w91) -> ("Ctrl"=w88:bool)
                n221 = case shown="\"Left\"" w90 {
                  tunnel: [_ w108 w112 "Action: Move Focus to Edit" ("State(s) in Front (\"\")")] -> w95
                  tunnel: w88 -> [_ w107 w111 _]
                  frame "ASCII", Default {
                  }
                  frame "Right" {
                    n222 = Select(t="Action: Move to Next Part\nAction: Update Current Range String\nUI: Update Candidate" ("State(s) in Front (\"\")"), s=w107, f="Action: Update Current Range String\nUI: Update Candidate" ("State(s) in Front (\"\")")) -> (s? t:f=w108:string)
                  }
                  frame "Left" {
                    n223 = Select(t="Action: Move to Previous Part\nAction: Update Current Range String\nUI: Update Candidate" ("State(s) in Front (\"\")"), s=w111, f="Action: Update Current Range String\nUI: Update Candidate" ("State(s) in Front (\"\")")) -> (s? t:f=w112:string)
                  }
                  frame "F2" {
                  }
                }
                n224 = case shown="49..57" w89 {
                  selector: w89 -> [_ w126]
                  tunnel: [_ w124] -> w94
                  tunnel: [_ TRUE] -> w105
                  frame 0, Default {
                  }
                  frame 49..57 {
                    n225 = Subtract(x=w126, y=i16 49) -> (x-y=w124:i16)
                  }
                }
                n226 = property on="Candidates" class="MCListbox (strict)"() -> ("ItemNames"=w103:string[][])  [unwired: 2 in, 2 out]
                n227 = And(x=w105, y=w88) -> (x .and. y?=w104:bool)
                n228 = Index Array(array=w103, index (row)=w94, index (col)=0 ("disabled index (col)")) -> (element=w99:string)
                n229 = Empty String/Path?(string/path=w99) -> (empty?=w101:bool)
                n230 = call <vilib>:"Add State(s) to Queue__JKI_lib_State_Machine.vi"("State(s) in Front (\"\")"=w95, "State(s) in (\"\")"=w93) -> ("States Out"=w96:string)  [unwired: 13 in]
                n231 = Not(x=w101) -> (.not. x?=w100:bool)
                n232 = And(x=w100, y=w104) -> (x .and. y?=w97:bool)
                n233 = case shown="True" w97 {
                  tunnel: w99 -> [_ w122]
                  tunnel: ["Action: Update Current Range String\nUI: Update Candidate" ("States Out") w119] -> w98
                  tunnel: w94 -> [_ w117]
                  frame False {
                  }
                  frame True {
                    n234 = call "CSM - Make String Arguments Safe.vi"("Argurment String"=w122) -> ("Safe Argurment String"=w118:string)  [unwired: 8 in]
                    n235 = local write "Candidates"(w117) -> ()
                    n236 = call <vilib>:"Build State String with Arguments__JKI_lib_State_Machine.vi"("Arguments (\"\")"=w118, "State"="Action: Replace Selction") -> ("State with Arguments"=w120:string)  [unwired: 4 in]
                    n237 = call <vilib>:"Add State(s) to Queue__JKI_lib_State_Machine.vi"("State(s) in (\"\")"=w120) -> ("States Out"=w119:string)  [unwired: 14 in]
                  }
                }
                n238 = call <vilib>:"Add State(s) to Queue__JKI_lib_State_Machine.vi"("State(s) in Front (\"\")"=w98, "State(s) in (\"\")"=w96) -> ("States Out"=w92:string)  [unwired: 13 in]
                n239 = event-data() -> ()  [unwired: 2 in, 1 out]
              }
            }
          }
          frame "Exit" {
            n240 = Unregister For Events(event registration refnum=w129) -> (error out=w128:errorcluster)  [unwired: 1 in]
            n241 = call <vilib>:"Clear Errors.vi"("error in (no error)"=w128) -> ()  [unwired: 5 in, 2 out]
          }
        }
      }
      n242 = Unbundle By Name(w14) -> ("CSM States"=w13:string)
    }
    frame Error {
    }
  }
  "Error out" <- w4
  "Command out" <- w1
